vi "Test1.vi"() -> ()   [LabVIEW 2020]
uses:
  <vilib>/gpm_packages/@cs/user-manager/Source/User Configuration Manager/User Configuration Manager.lvclass
  C:/Program Files/National Instruments/LabVIEW 2020/vi.lib/gpm_packages/@cs/user-manager/Source/iUser Configuration Manager/iUser Configuration Manager.lvclass
  <vilib>/gpm_packages/@cs/user-manager/Source/SHA-1 Encryption/SHA-1.lvclass
  C:/Program Files/National Instruments/LabVIEW 2020/vi.lib/gpm_packages/@cs/user-manager/Source/iEncryption/iEncryption.lvclass
  <vilib>/gpm_packages/@cs/persistence/source/CAML/CAML.lvclass
  C:/Program Files/National Instruments/LabVIEW 2020/vi.lib/gpm_packages/@cs/persistence/source/IPersist/IPersist.lvclass
  <vilib>/gpm_packages/@cs/persistence/source/XML/XML.lvclass
  <vilib>/gpm_packages/@cs/user-manager/Source/User Configuration Manager Ref/By Ref.lvlib
panel:
  out "error out 2":errorcluster
  out "error out":errorcluster
  out "Users":string[](array[string])
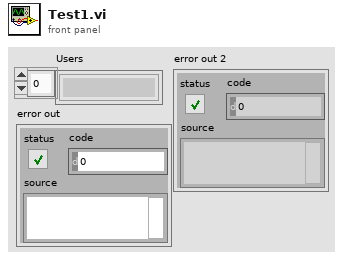
[diagram p1: front panel]
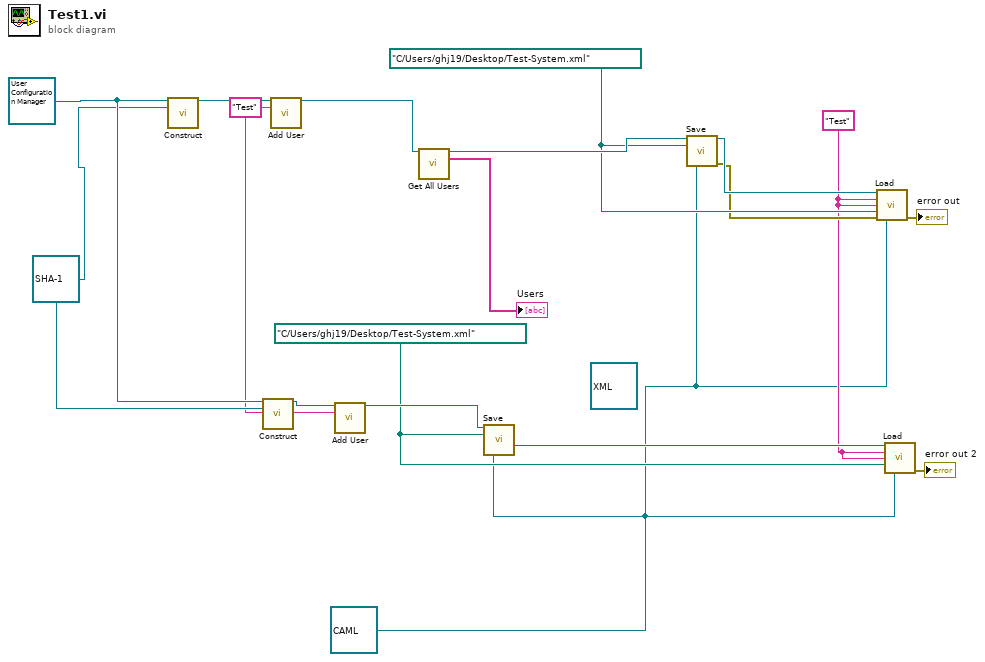
[diagram p0: block diagram]
diagram:
  w1 = refnum<class "CAML.lvclass"> refnum ("CAML.lvlib:CAML.lvclass")
  w4 = path "C:/Users/ghj19/Desktop/Test-System.xml" ("Path")
  w3 = "Test" ("Username")
  w13 = path "C:/Users/ghj19/Desktop/Test-System.xml" ("Path")
  (unwired) refnum<class "XML.lvclass"> refnum ("XML.lvlib:XML.lvclass")
  w7 = "Test" ("Username")
  w9 = refnum<class "SHA-1.lvclass"> refnum ("User Configuration Manager.lvlib:SHA-1.lvclass")
  w10 = refnum<class "User Configuration Manager.lvclass"> refnum ("User Configuration Manager.lvlib:User Configuration Manager")
  n1 = call <vilib>:"Construct.vi"("iUser Configuration Manager in"=w10, "Encryption Type"=w9) -> ("dup iUser Configuration Manager DVR"=w18:refnum<data-value>)  [unwired: 12 in, 1 out]
  n2 = call-dynamic <vilib>:"Construct.vi"("User Configuration Manager in"=w10, "Encryption Type"=w9) -> ("User Configuration Manager out"=w8:refnum<class "User Configuration Manager.lvclass">)  [unwired: 12 in, 1 out]
  n3 = call <vilib>:"Add User.vi"("iUser Configuration Manager DVR"=w18, "Username"=w7) -> ("dup iUser Configuration Manager DVR"=w17:refnum<data-value>)  [unwired: 11 in, 2 out]
  n4 = call-dynamic <vilib>:"Add User.vi"("User Configuration Manager in"=w8, "Username"=w7) -> ("User Configuration Manager out"=w6:refnum<class "User Configuration Manager.lvclass">)  [unwired: 11 in, 2 out]
  n5 = call <vilib>:"Get All Users.vi"("iUser Configuration Manager DVR"=w17) -> ("dup iUser Configuration Manager DVR"=w15:refnum<data-value>, "Users"=→"Users":string[])  [unwired: 11 in, 2 out]
  n6 = call-dynamic <vilib>:"Save.vi"("User Configuration Manager in"=w6, "Path"=w4, "Persistence"=w1) -> ("User Configuration Manager out"=w5:refnum<class "User Configuration Manager.lvclass">)  [unwired: 11 in, 1 out]
  n7 = call <vilib>:"Save.vi"("iUser Configuration Manager DVR"=w15, "Path"=w13, "Persistence"=w1) -> ("dup iUser Configuration Manager DVR"=w14:refnum<data-value>, "error out"=w11:errorcluster)  [unwired: 11 in]
  n8 = call <vilib>:"Load.vi"("iUser Configuration Manager DVR"=w14, "Username"=w3, "Password"=w3, "Path"=w13, "error in"=w11, "Persistence"=w1) -> ("error out"=→"error out":errorcluster)  [unwired: 6 in, 3 out]
  n9 = call-dynamic <vilib>:"Load.vi"("User Configuration Manager"=w5, "Username"=w3, "Password"=w3, "Path"=w4, "Persistence"=w1) -> ("error out"=→"error out 2":errorcluster)  [unwired: 7 in, 3 out]
